vi "Get Request example.vi"() -> ()   [LabVIEW 2016]
panel:
  out "data":T1(array[cluster])
  in  "Team":T2(ring)
  in  "error in (no error)":errorcluster
  out "error out":errorcluster
  in  "Authentication Info":T3={"Client ID"="", "Client Secret"="", "Redirect URI"="", "Token Endpoint"="https://app.asana.com/-/oauth_token", "Scope"=""}
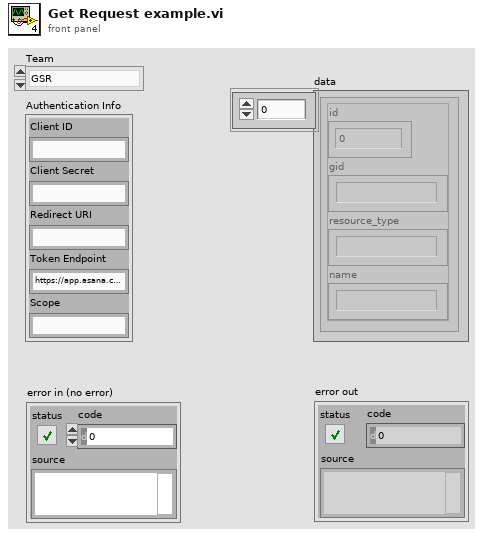
[diagram p1: front panel]
types:
  T1 = cluster{"id":i32, "gid":string, "resource_type":string, "name":string}[]
  T2 = enum16{"GSR", "Research Projects", "Undergrads", "Researchers", "Hardware", "Software", "LevyLab", "Samples", "Manuscripts", "AoT", "WorkStudy"}
  T3 = cluster{"Client ID":string, "Client Secret":string, "Redirect URI":string, "Token Endpoint":string, "Scope":string}
  T4 = typedef "REST Client.lvlib/REST Client.lvclass/HTTP Header.ctl" = cluster{"header":string, "value":string}
  T5 = cluster{"id":i32, "gid":string, "name":string, "resource_type":string}[]
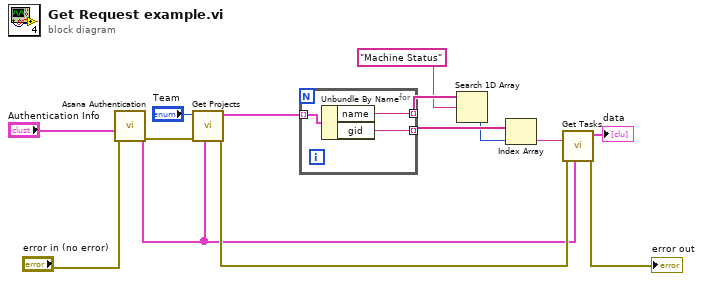
[diagram p0: block diagram]
diagram:
  n1 = call "Asana Authentication.vi"("error in (no error)"="error in (no error)", "Authentication Info"="Authentication Info") -> ("error out"=w13:errorcluster, "Authentication Header"=w2:T4[])  [unwired: 6 in, 2 out]
  n2 = call "Get Projects.vi"("Authorization"=w2, "error in (no error)"=w13, "Team"="Team") -> ("error out"=w5:errorcluster, "Projects Out"=w1:T5)  [unwired: 7 in]
  n3 = for {
    tunnel: w1 -> [w17] mode=indexing
    tunnel: [w16] -> w8 mode=indexing
    tunnel: [w15] -> w10 mode=indexing
    n4 = Unbundle By Name(w17) -> ("name"=w16:string, "gid"=w15:string)
  }
  n5 = Search 1D Array(1D array=w8, element="Machine Status") -> (index of element=w9:i32)  [unwired: 1 in]
  n6 = Index Array(array=w10, index=w9) -> (element=w6:string)
  n7 = call "Get Tasks.vi"("Authorization"=w2, "error in (no error)"=w5, "Project GID"=w6) -> ("error out"=→"error out":errorcluster, "Tasks Out"=→"data":T1)  [unwired: 7 in]
